vi "_31_Sample_qsns_9[7].vi"() -> ()   [LabVIEW 2020]
panel:
  out "XY Graph":cluster{"Y":dbl[], "Y":dbl[]}[](graph)
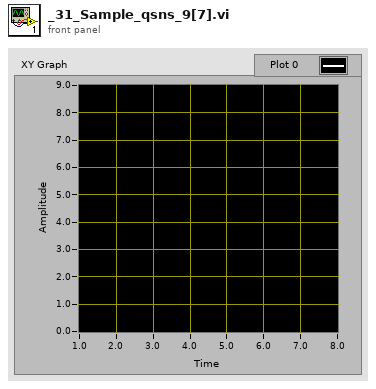
[diagram p1: front panel]
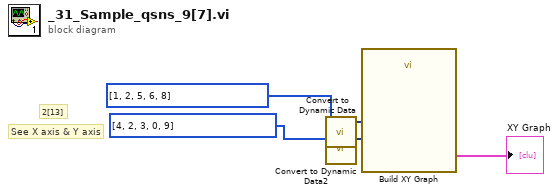
[diagram p0: block diagram]
diagram:
  # "See X axis & Y axis"
  # "2[13]"
  n1 = call "Convert to Dynamic Data"("Array"=i32[] [1, 2, 5, 6, 8]) -> ("Dynamic Data Type"=w3:dynamicdata)  [unwired: 3 in]
  n2 = call "Convert to Dynamic Data2"("Array"=i32[] [4, 2, 3, 0, 9]) -> ("Dynamic Data Type"=w1:dynamicdata)  [unwired: 3 in]
  n3 = call "Build XY Graph"("Y Input"=w1, "X Input"=w3) -> ("XY Graph"=→"XY Graph":cluster{"X":dbl[], "Y":dbl[]}[])  [unwired: 8 in, 1 out]
